vi "Terminal-Alert-PressureSystem.vi"(11 "液压子系统设备信息":T1) -> (3 "液压子系统设备信息输出":T1)   [LabVIEW 2014]
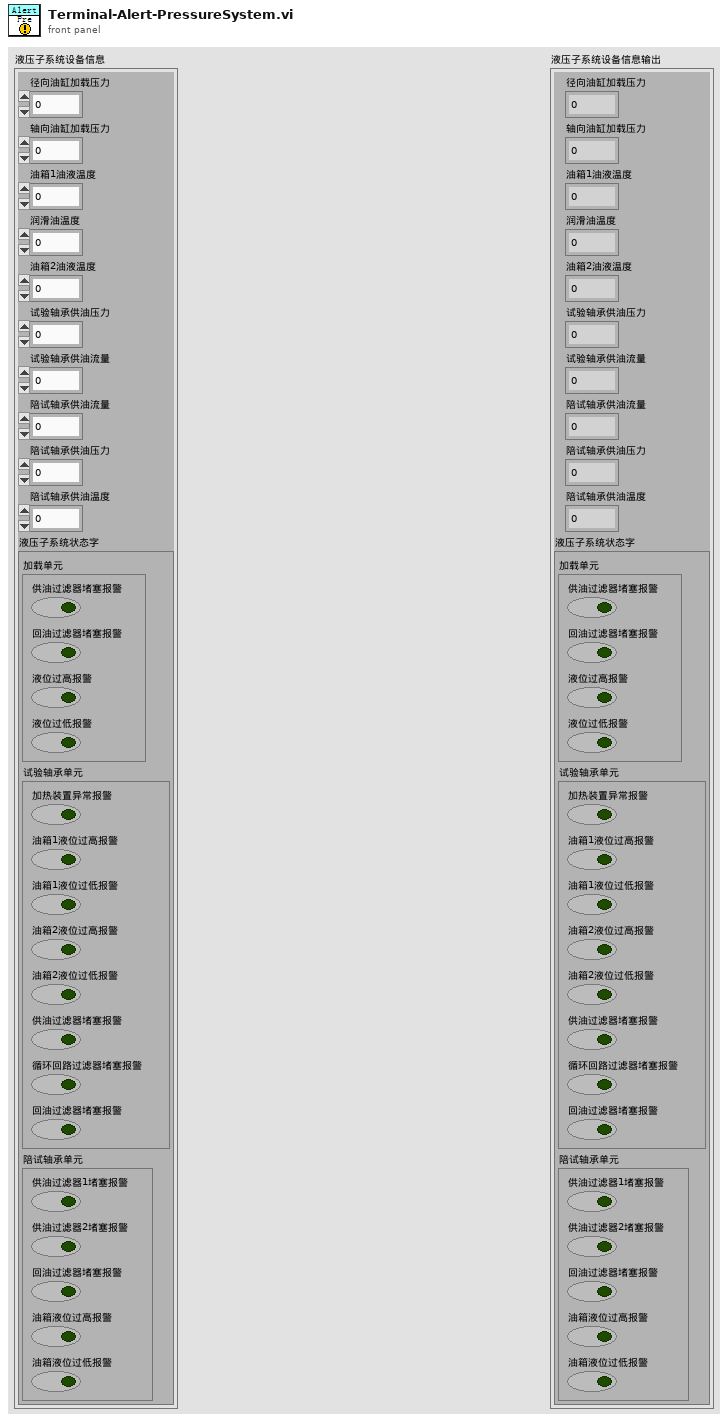
[diagram p1: front panel]
types:
  T1 = cluster{"径向油缸加载压力":u16, "轴向油缸加载压力":u16, "油箱1油液温度":u16, "润滑油温度":u16, "油箱2油液温度":u16, "试验轴承供油压力":u16, "试验轴承供油流量":u16, "陪试轴承供油流量":u16, "陪试轴承供油压力":u16, "陪试轴承供油温度":u16, "液压子系统状态字":cluster{"加载单元":cluster{"供油过滤器堵塞报警":bool, "回油过滤器堵塞报警":bool, "液位过高报警":bool, "液位过低报警":bool}, "试验轴承单元":cluster{"加热装置异常报警":bool, "油箱1液位过高报警":bool, "油箱1液位过低报警":bool, "油箱2液位过高报警":bool, "油箱2液位过低报警":bool, "供油过滤器堵塞报警":bool, "循环回路过滤器堵塞报警":bool, "回油过滤器堵塞报警":bool}, "陪试轴承单元":cluster{"供油过滤器1堵塞报警":bool, "供油过滤器2堵塞报警":bool, "回油过滤器堵塞报警":bool, "油箱液位过高报警":bool, "油箱液位过低报警":bool}}}
  T2 = cluster{"报警级别":string, "报警系统":string, "报警详情":string, "备注":string}
  T3 = cluster{"加载单元":cluster{"供油过滤器堵塞报警":bool, "回油过滤器堵塞报警":bool, "液位过高报警":bool, "液位过低报警":bool}, "试验轴承单元":cluster{"加热装置异常报警":bool, "油箱1液位过高报警":bool, "油箱1液位过低报警":bool, "油箱2液位过高报警":bool, "油箱2液位过低报警":bool, "供油过滤器堵塞报警":bool, "循环回路过滤器堵塞报警":bool, "回油过滤器堵塞报警":bool}, "陪试轴承单元":cluster{"供油过滤器1堵塞报警":bool, "供油过滤器2堵塞报警":bool, "回油过滤器堵塞报警":bool, "油箱液位过高报警":bool, "油箱液位过低报警":bool}}
  T4 = cluster{"供油过滤器堵塞报警":bool, "回油过滤器堵塞报警":bool, "液位过高报警":bool, "液位过低报警":bool}
  T5 = cluster{"加热装置异常报警":bool, "油箱1液位过高报警":bool, "油箱1液位过低报警":bool, "油箱2液位过高报警":bool, "油箱2液位过低报警":bool, "供油过滤器堵塞报警":bool, "循环回路过滤器堵塞报警":bool, "回油过滤器堵塞报警":bool}
  T6 = cluster{"供油过滤器1堵塞报警":bool, "供油过滤器2堵塞报警":bool, "回油过滤器堵塞报警":bool, "油箱液位过高报警":bool, "油箱液位过低报警":bool}
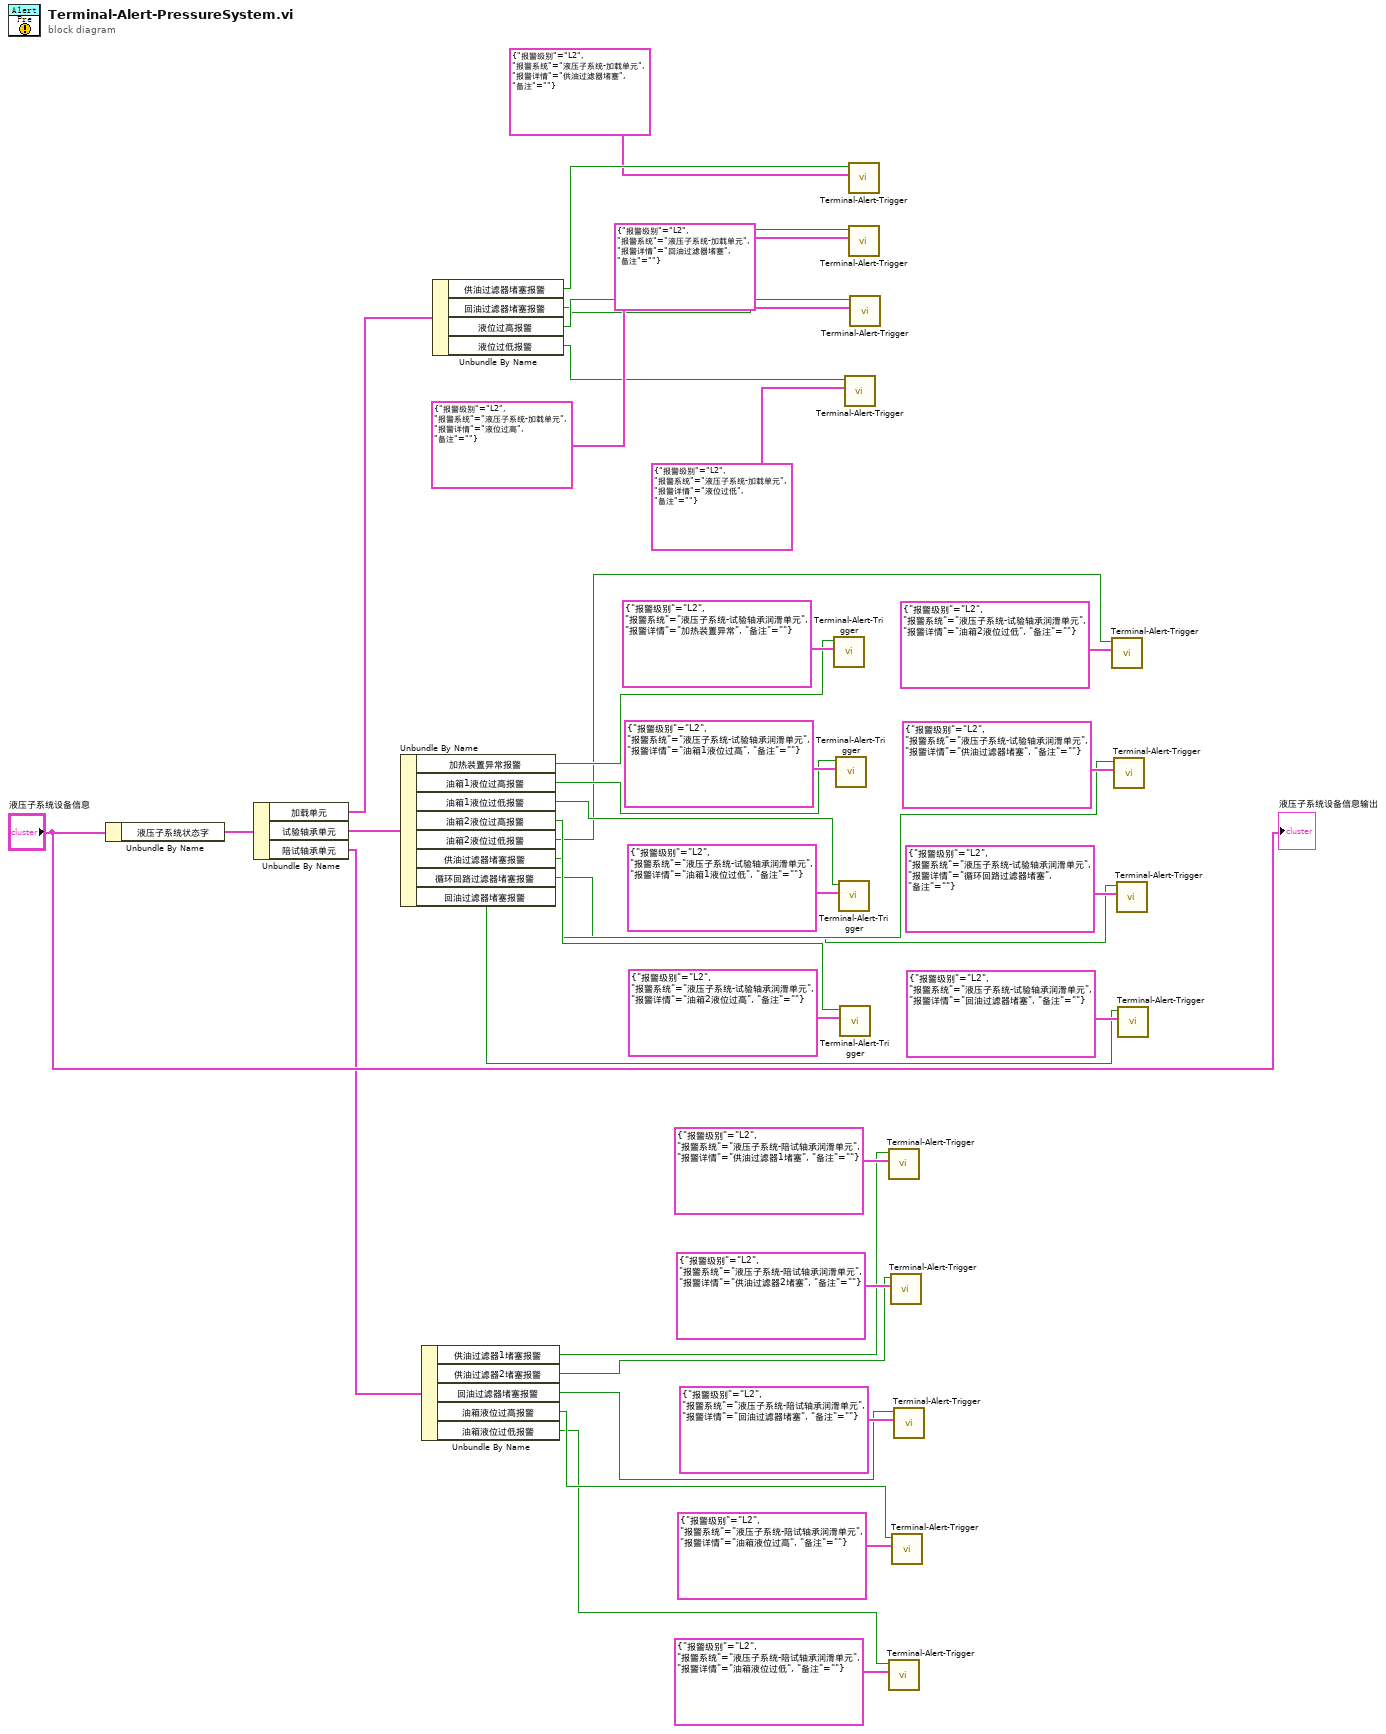
[diagram p0: block diagram]
diagram:
  n1 = Unbundle By Name("液压子系统设备信息") -> ("液压子系统状态字"=w38:T3)
  n2 = Unbundle By Name(w38) -> ("加载单元"=w37:T4, "试验轴承单元"=w36:T5, "陪试轴承单元"=w35:T6)
  n3 = Unbundle By Name(w36) -> ("加热装置异常报警"=w18:bool, "油箱1液位过高报警"=w17:bool, "油箱1液位过低报警"=w16:bool, "油箱2液位过高报警"=w15:bool, "油箱2液位过低报警"=w14:bool, "供油过滤器堵塞报警"=w13:bool, "循环回路过滤器堵塞报警"=w12:bool, "回油过滤器堵塞报警"=w11:bool)
  n4 = Unbundle By Name(w35) -> ("供油过滤器1堵塞报警"=w5:bool, "供油过滤器2堵塞报警"=w4:bool, "回油过滤器堵塞报警"=w3:bool, "油箱液位过高报警"=w2:bool, "油箱液位过低报警"=w1:bool)
  n5 = Unbundle By Name(w37) -> ("供油过滤器堵塞报警"=w34:bool, "回油过滤器堵塞报警"=w27:bool, "液位过高报警"=w28:bool, "液位过低报警"=w29:bool)
  n6 = call "Terminal-Alert-Trigger.vi"("报警信息"=T2 {"报警级别"="L2", "报警系统"="液压子系统-试验轴承润滑单元", "报警详情"="加热装置异常", "备注"=""}, "是否触发(T)"=w18) -> ()  [unwired: 9 in, 1 out]
  n7 = call "Terminal-Alert-Trigger.vi"("报警信息"=T2 {"报警级别"="L2", "报警系统"="液压子系统-试验轴承润滑单元", "报警详情"="油箱1液位过高", "备注"=""}, "是否触发(T)"=w17) -> ()  [unwired: 9 in, 1 out]
  n8 = call "Terminal-Alert-Trigger.vi"("报警信息"=T2 {"报警级别"="L2", "报警系统"="液压子系统-试验轴承润滑单元", "报警详情"="油箱1液位过低", "备注"=""}, "是否触发(T)"=w16) -> ()  [unwired: 9 in, 1 out]
  n9 = call "Terminal-Alert-Trigger.vi"("报警信息"=T2 {"报警级别"="L2", "报警系统"="液压子系统-试验轴承润滑单元", "报警详情"="油箱2液位过高", "备注"=""}, "是否触发(T)"=w15) -> ()  [unwired: 9 in, 1 out]
  n10 = call "Terminal-Alert-Trigger.vi"("报警信息"=T2 {"报警级别"="L2", "报警系统"="液压子系统-加载单元", "报警详情"="液位过低", "备注"=""}, "是否触发(T)"=w29) -> ()  [unwired: 9 in, 1 out]
  n11 = call "Terminal-Alert-Trigger.vi"("报警信息"=T2 {"报警级别"="L2", "报警系统"="液压子系统-加载单元", "报警详情"="供油过滤器堵塞", "备注"=""}, "是否触发(T)"=w34) -> ()  [unwired: 9 in, 1 out]
  n12 = call "Terminal-Alert-Trigger.vi"("报警信息"=T2 {"报警级别"="L2", "报警系统"="液压子系统-加载单元", "报警详情"="回油过滤器堵塞", "备注"=""}, "是否触发(T)"=w27) -> ()  [unwired: 9 in, 1 out]
  n13 = call "Terminal-Alert-Trigger.vi"("报警信息"=T2 {"报警级别"="L2", "报警系统"="液压子系统-加载单元", "报警详情"="液位过高", "备注"=""}, "是否触发(T)"=w28) -> ()  [unwired: 9 in, 1 out]
  n14 = call "Terminal-Alert-Trigger.vi"("报警信息"=T2 {"报警级别"="L2", "报警系统"="液压子系统-陪试轴承润滑单元", "报警详情"="供油过滤器1堵塞", "备注"=""}, "是否触发(T)"=w5) -> ()  [unwired: 9 in, 1 out]
  n15 = call "Terminal-Alert-Trigger.vi"("报警信息"=T2 {"报警级别"="L2", "报警系统"="液压子系统-陪试轴承润滑单元", "报警详情"="油箱液位过低", "备注"=""}, "是否触发(T)"=w1) -> ()  [unwired: 9 in, 1 out]
  n16 = call "Terminal-Alert-Trigger.vi"("报警信息"=T2 {"报警级别"="L2", "报警系统"="液压子系统-陪试轴承润滑单元", "报警详情"="供油过滤器2堵塞", "备注"=""}, "是否触发(T)"=w4) -> ()  [unwired: 9 in, 1 out]
  n17 = call "Terminal-Alert-Trigger.vi"("报警信息"=T2 {"报警级别"="L2", "报警系统"="液压子系统-陪试轴承润滑单元", "报警详情"="油箱液位过高", "备注"=""}, "是否触发(T)"=w2) -> ()  [unwired: 9 in, 1 out]
  n18 = call "Terminal-Alert-Trigger.vi"("报警信息"=T2 {"报警级别"="L2", "报警系统"="液压子系统-陪试轴承润滑单元", "报警详情"="回油过滤器堵塞", "备注"=""}, "是否触发(T)"=w3) -> ()  [unwired: 9 in, 1 out]
  n19 = call "Terminal-Alert-Trigger.vi"("报警信息"=T2 {"报警级别"="L2", "报警系统"="液压子系统-试验轴承润滑单元", "报警详情"="油箱2液位过低", "备注"=""}, "是否触发(T)"=w14) -> ()  [unwired: 9 in, 1 out]
  n20 = call "Terminal-Alert-Trigger.vi"("报警信息"=T2 {"报警级别"="L2", "报警系统"="液压子系统-试验轴承润滑单元", "报警详情"="供油过滤器堵塞", "备注"=""}, "是否触发(T)"=w13) -> ()  [unwired: 9 in, 1 out]
  n21 = call "Terminal-Alert-Trigger.vi"("报警信息"=T2 {"报警级别"="L2", "报警系统"="液压子系统-试验轴承润滑单元", "报警详情"="循环回路过滤器堵塞", "备注"=""}, "是否触发(T)"=w12) -> ()  [unwired: 9 in, 1 out]
  n22 = call "Terminal-Alert-Trigger.vi"("报警信息"=T2 {"报警级别"="L2", "报警系统"="液压子系统-试验轴承润滑单元", "报警详情"="回油过滤器堵塞", "备注"=""}, "是否触发(T)"=w11) -> ()  [unwired: 9 in, 1 out]
  "液压子系统设备信息输出" <- "液压子系统设备信息"
